vi "ManipWait.vi"(2 "Reinit":bool, 3 "Instruction String":string) -> (0 "Error Out":errorcluster, 1 "Advance Trigger":bool)   [LabVIEW 2019]
doc: "This VI pauses the subsystem sequencer until the specified condition is met. Six different modes are available: time_delay, drive_step, dist_from_start, dist_from_end, time_since_shooter, and balls_shot.\n\nParameters:\ntime_delay --> wait for param1{time delay (ms)} or if -1 from the dashboard (s), param2{1}\ndrive_step --> wait for param1{drivesequence step (#)}, param2{1}\ndist_from_start --> wait for param1{distance (in)} from start of current path, param2{1}\ndist_from_end --> wait for param1{distance (in)} from end of current path, param2{1}\ntime_since_shooter --> wait for param1{time (ms)} since shooter started shooting, param2{1}\nballs_shot --> wait for param2{current balls shot}, or until param1{timeout(ms), or set to -1 to ignore}"
uses:
  SafeParser_Integer.vi
  SafeParser_Float.vi
  SafeParser_String.vi
  dsdata.vi
  autoninfo.vi
  sensors.vi
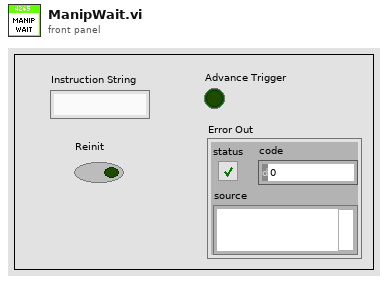
[diagram p1: front panel]
types:
  T1 = enum16{"Center", "North", "NorthWest", "West", "SouthWest", "South", "SouthEast", "East", "NorthEast"}
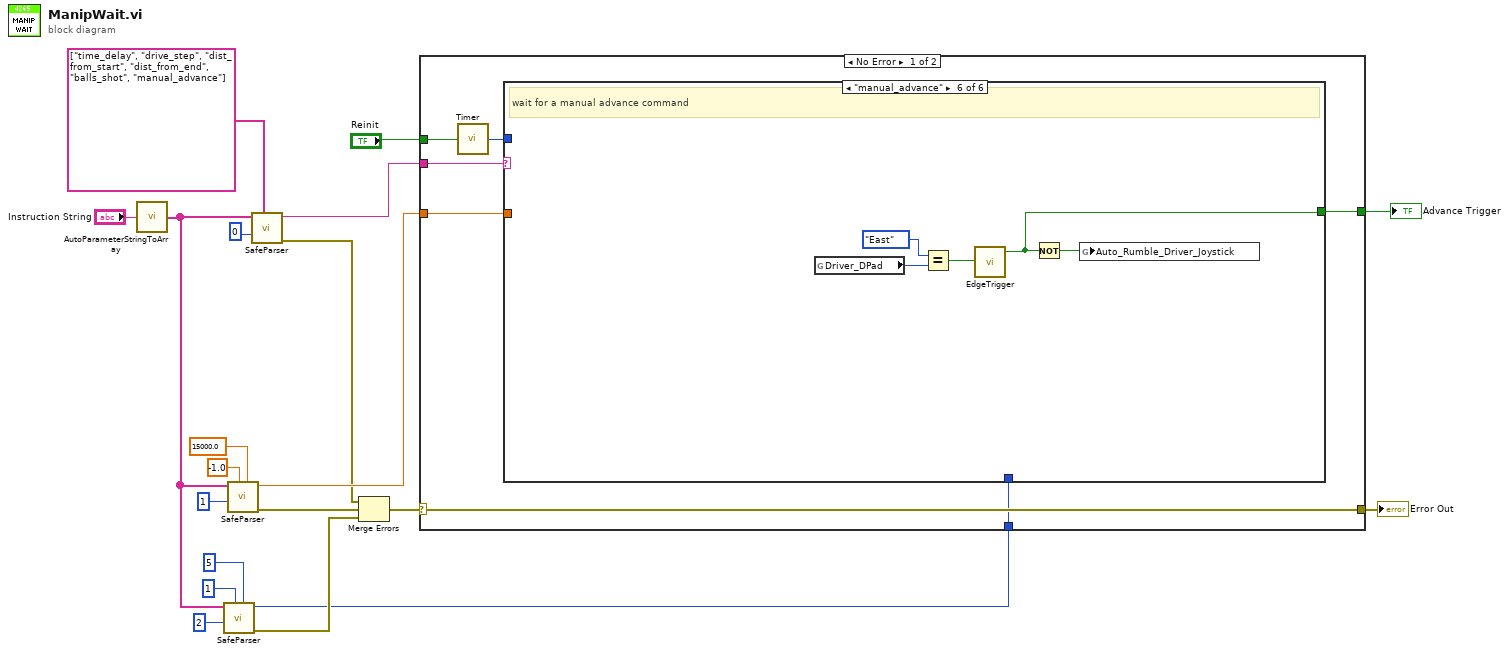
[diagram p0: block diagram]
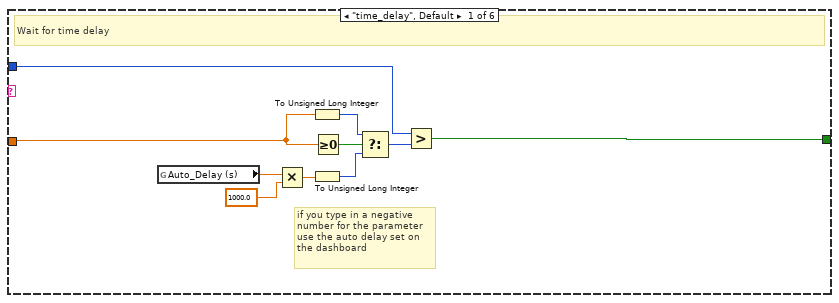
[diagram p2: hidden frame]
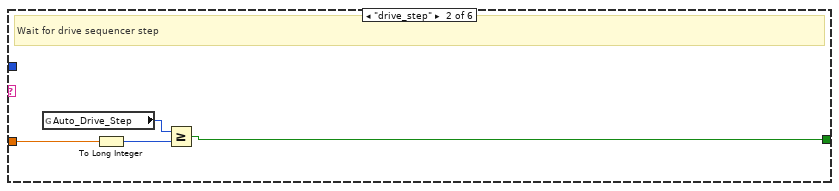
[diagram p3: hidden frame]
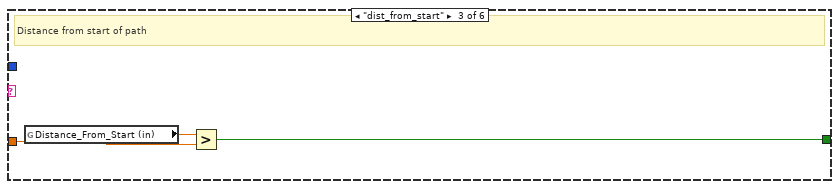
[diagram p4: hidden frame]
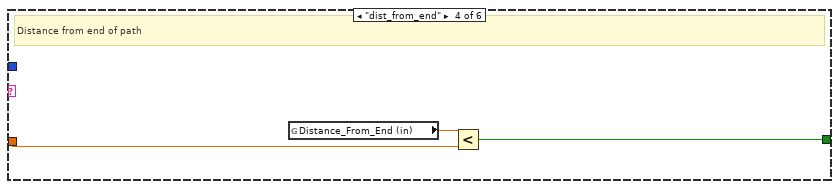
[diagram p5: hidden frame]
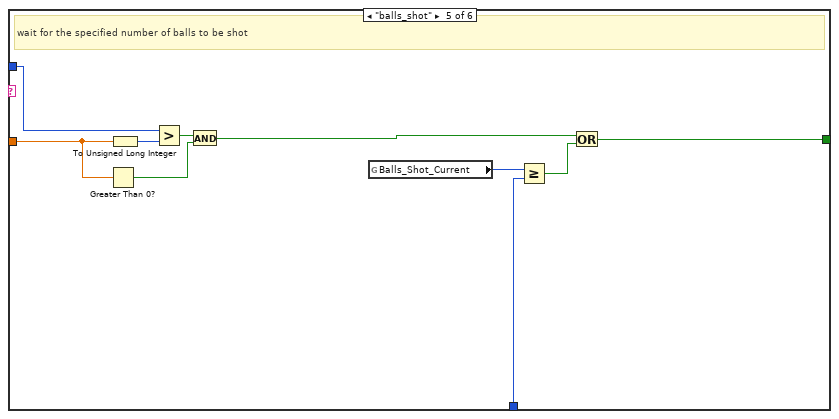
[diagram p6: hidden frame]
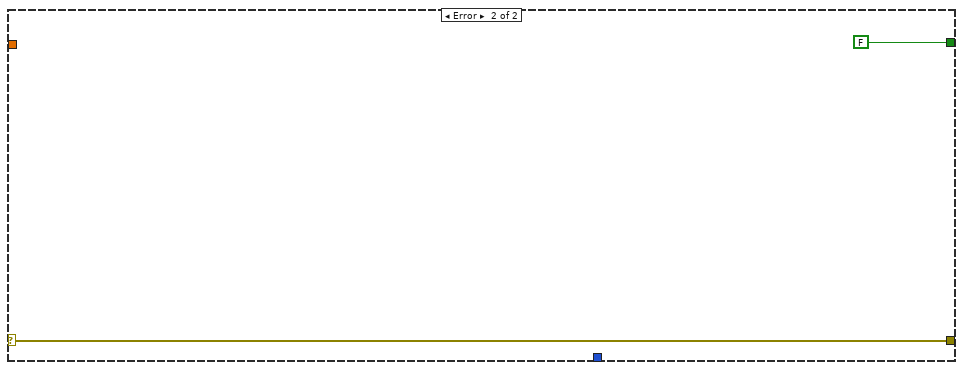
[diagram p7: hidden frame]
diagram:
  n1 = call "AutoParameterStringToArray.vi"("Parameter String"="Instruction String") -> ("Parsed Parameters"=w7:string[])
  n2 = call-poly "SafeParser.vi"("Maximum"=5, "Minimum"=1, "Array Index"=2 ("Parameter Index"), "String Array"=w7) -> ("Error Out"=w6:errorcluster, "Typecast  Value"=w5:i32)  [unwired: 6 in]
  n3 = call-poly "SafeParser.vi"("Maximum"=15000.0, "Minimum"=-1.0, "Array Index"=1 ("Parameter Index"), "String Array"=w7) -> ("Error Out"=w10:errorcluster, "Typecast  Value"=w13:dbl)  [unwired: 6 in]
  n4 = call-poly "SafeParser.vi"("Allowed Values"=string[] ["time_delay", "drive_step", "dist_from_start", "dist_from_end", "balls_shot", "manual_advance"], "Array Index"=0 ("Parameter Index"), "String Array"=w7) -> ("Error Out"=w9:errorcluster, "Typecast Value"=w11:string)  [unwired: 7 in]
  n5 = Merge Errors(w9, w10, w6) -> (w14:errorcluster)
  n6 = case shown="No Error" w14 {
    selector: w14 -> [w25 w63]
    tunnel: w11 -> [w27 _]
    tunnel: [w26 FALSE] -> w20
    tunnel: [w25 w63] -> w19
    tunnel: w13 -> [w24 _]
    tunnel: w5 -> [w23 _]
    tunnel: "Reinit" -> [w21 _]
    frame No Error {
      n7 = call "Timer.vi"("Reset Timer"=w21) -> ("Time (ms)"=w22:u32)
      n8 = case shown="\"manual_advance\"" w27 {
        tunnel: w22 -> [w30 _ _ _ w54 _]
        tunnel: [w29 w39 w44 w47 w48 w58] -> w26
        tunnel: w24 -> [w28 w38 w42 w45 w53 _]
        tunnel: w23 -> [_ _ _ _ w56 _]
        frame "time_delay", Default {
          # "if you type in a negative\nnumber for the parameter\nuse the auto delay set on \nthe dashboard"
          # "Wait for time delay"
          n9 = global read "dsdata.vi" "Auto_Delay (s)"() -> (w35:dbl)
          n10 = Multiply(x=w35, y=1000.0) -> (x*y=w36:dbl)
          n11 = To Unsigned Long Integer(number=w28) -> (unsigned 32bit integer=w34:u32)
          n12 = To Unsigned Long Integer(number=w36) -> (unsigned 32bit integer=w37:u32)
          n13 = Greater Or Equal To 0?(x=w28) -> (x >= 0?=w33:bool)
          n14 = Select(t=w34, s=w33, f=w37) -> (s? t:f=w31:u32)
          n15 = Greater?(x=w30, y=w31) -> (0:w29:bool)
        }
        frame "drive_step" {
          # "Wait for drive sequencer step"
          n16 = global read "autoninfo.vi" "Auto_Drive_Step"() -> (w41:i32)
          n17 = To Long Integer(number=w38) -> (32bit integer=w40:i32)
          n18 = Greater Or Equal?(x=w41, y=w40) -> (x >= y?=w39:bool)
        }
        frame "dist_from_start" {
          # "Distance from start of path"
          n19 = global read "autoninfo.vi" "Distance_From_Start (in)"() -> (w43:dbl)
          n20 = Greater?(x=w43, y=w42) -> (0:w44:bool)
        }
        frame "dist_from_end" {
          # "Distance from end of path"
          n21 = global read "autoninfo.vi" "Distance_From_End (in)"() -> (w46:dbl)
          n22 = Less?(x=w46, y=w45) -> (x < y?=w47:bool)
        }
        frame "balls_shot" {
          # "wait for the specified number of balls to be shot"
          n23 = Greater Than 0?(x=w53) -> (x > 0?=w51:bool)
          n24 = To Unsigned Long Integer(number=w53) -> (unsigned 32bit integer=w55:u32)
          n25 = Greater?(x=w54, y=w55) -> (0:w52:bool)
          n26 = And(x=w52, y=w51) -> (x .and. y?=w49:bool)
          n27 = global read "sensors.vi" "Balls_Shot_Current"() -> (w57:i32)
          n28 = Greater Or Equal?(x=w57, y=w56) -> (x >= y?=w50:bool)
          n29 = Or(x=w49, y=w50) -> (x .or. y?=w48:bool)
        }
        frame "manual_advance" {
          # "wait for a manual advance command"
          n30 = global read "dsdata.vi" "Driver_DPad"() -> (w62:T1)
          n31 = Equal?(x=T1."East" ("Driver_DPad"), y=w62) -> (x = y?=w59:bool)
          n32 = call "EdgeTrigger.vi"("Input Signal"=w59) -> ("Rising Edge Trigger"=w58:bool)  [unwired: 2 out]
          n33 = Not(x=w58) -> (.not. x?=w60:bool)
          n34 = global write "autoninfo.vi" "Auto_Rumble_Driver_Joystick"(w60) -> ()
        }
      }
    }
    frame Error {
    }
  }
  "Advance Trigger" <- w20
  "Error Out" <- w19
